vi "theta_calibration.vi"(6 "error in (no error)":errorcluster, 9 "log to file":path=path "C:/Users/tuphe10-memsbuddy/Desktop/test_VTI_theta_cal/test.txt", 11 "VISA Gaussmeter":refnum<visa-resource-name>="GPIB1::11::INSTR") -> (4 "error out":errorcluster, 5 "VISA resource name":refnum<visa-resource-name>)   [LabVIEW 2013]
uses:
  devices/gaussmeter/gaussmeter channels.ctl
panel:
  out "Channel 3":dbl format="%.2f"
  in  "channel 3":T1=enum."Z"
  out "Channel 3":cluster{dbl, dbl}[](graph)
  out "current theta (deg)":dbl format="%#_13g"
  in  "start theta (deg)":dbl format="%#_13g"
  in  "final theta (deg)":dbl=190.0 format="%#_13g"
  in  "increment (deg)":dbl=0.5 format="%#_13g"
  in  "channel 2":T1=enum."Y"
  in  "channel 1":T1
  out "Channel 2":cluster{dbl, "magnetic field (T)":dbl}[](graph)
  out "Channel 1":cluster{dbl, dbl}[](graph)
  out "Channel 2":dbl format="%.2f"
  out "Channel 1":dbl format="%.2f"
  # "This .vi sets the motor to 0deg (reference switch) & performs a user-defined turn while measuring field components with the Gaussmeter. It saves the data into a .txt file."
  # "NEVER exceed 320° !!!\nUse only positive values here!"
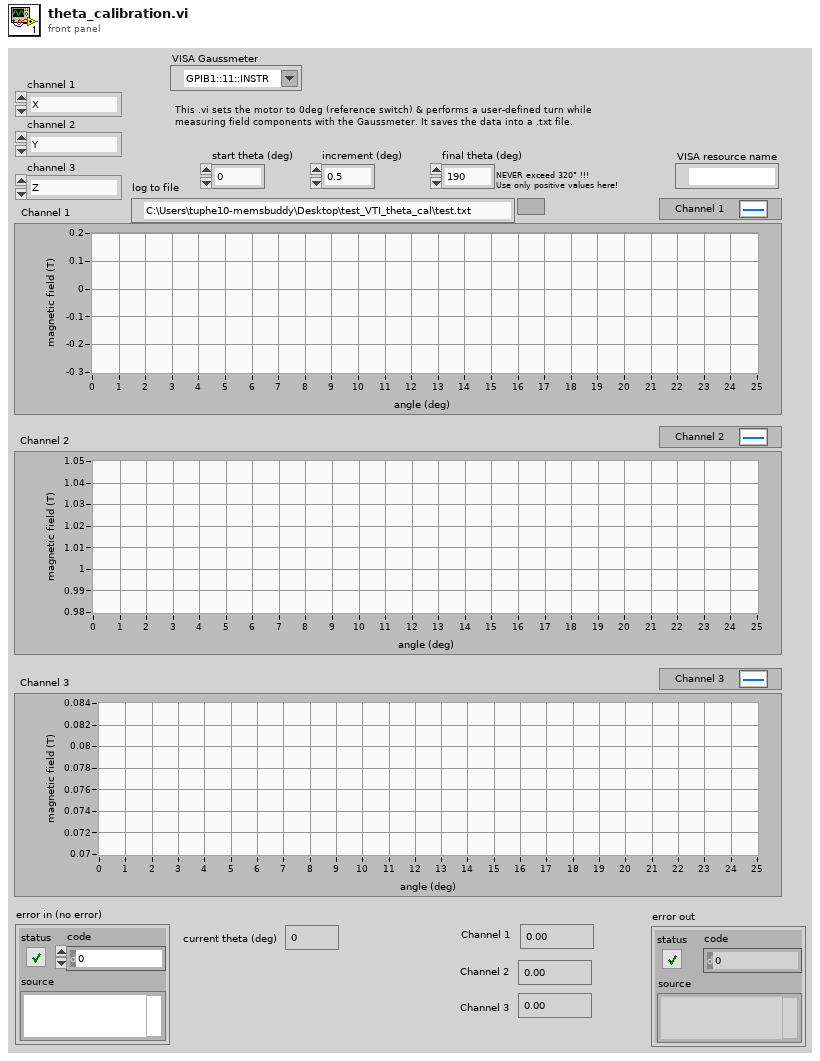
[diagram p1: front panel]
types:
  T1 = typedef "gaussmeter channels.ctl" = enum16{"X", "Y", "Z", "Vec"}
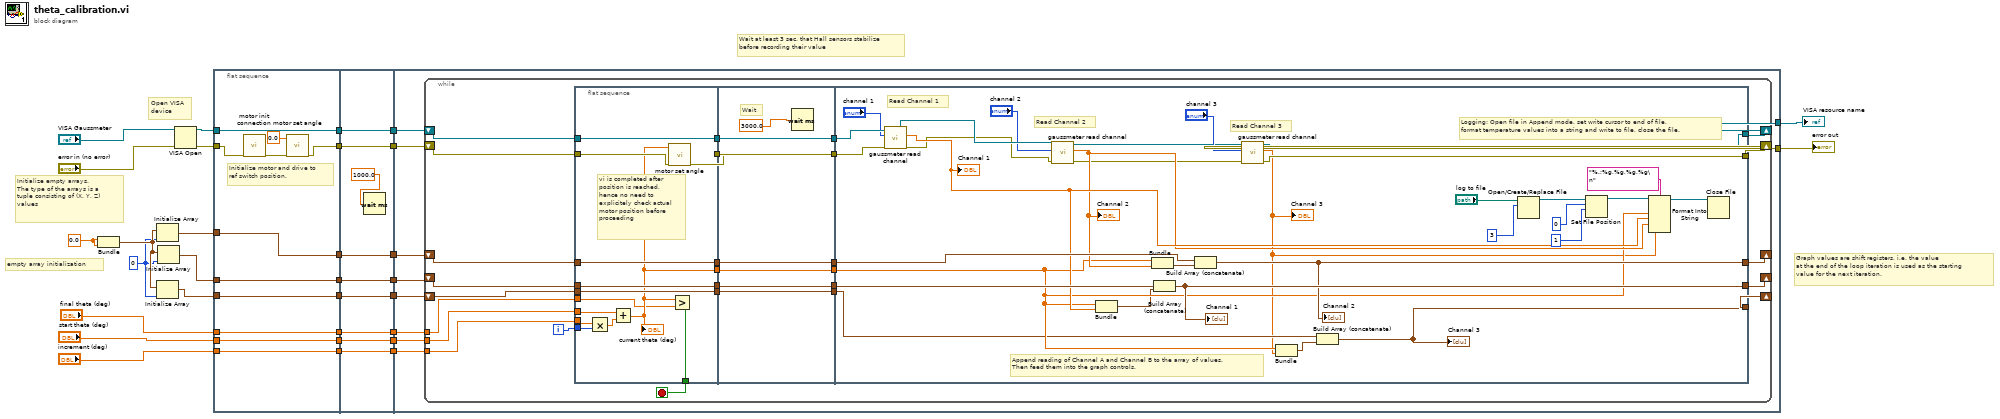
[diagram p0: block diagram]
diagram:
  w4 = 0
  w6 = 0.0
  # "Wait at least 3 sec. that Hall sensors stabilize\nbefore recording their value"
  # "empty array initialization"
  # "Graph values are shift registers, i.e. the value\nat the end of the loop iteration is used as the starting\nvalue for the next iteration."
  # "Initialize empty arrays.\nThe type of the arrays is a tuple consisting of (X, Y, Z) values"
  # "Open VISA\ndevice"
  n1 = Bundle(w6, w6) -> (w5:cluster{dbl, dbl})  [unwired: 1 in]
  n2 = Initialize Array(w5, w4) -> (w27:cluster{dbl, dbl}[])
  n3 = Initialize Array(w5, w4) -> (w2:cluster{dbl, dbl}[])
  n4 = Initialize Array(w5, w4) -> (w26:cluster{dbl, dbl}[])
  n5 = VISA Open(error in (no error)="error in (no error)", VISA resource name="VISA Gaussmeter") -> (VISA resource name=w29:refnum<visa-resource-name>, error out=w28:errorcluster)  [unwired: 3 in]
  n6 = flat-sequence {
    tunnel: "start theta (deg)" -> [w37]
    tunnel: "final theta (deg)" -> [w38]
    tunnel: "increment (deg)" -> [w39]
    tunnel: w26 -> [w40]
    tunnel: w27 -> [w41]
    tunnel: w28 -> [w34]
    tunnel: w29 -> [w42]
    tunnel: [w42] -> w20
    tunnel: [w33] -> w18
    tunnel: [w41] -> w16
    tunnel: [w40] -> w14
    tunnel: [w39] -> w12
    tunnel: [w38] -> w10
    tunnel: [w37] -> w8
    tunnel: [w32] -> w3
    tunnel: w2 -> [w32]
    tunnel: w20 -> [w51]
    tunnel: [w51] -> w19
    tunnel: w18 -> [w50]
    tunnel: [w50] -> w17
    tunnel: w16 -> [w49]
    tunnel: [w49] -> w15
    tunnel: w14 -> [w48]
    tunnel: [w48] -> w13
    tunnel: w12 -> [w47]
    tunnel: [w47] -> w11
    tunnel: w10 -> [w46]
    tunnel: [w46] -> w9
    tunnel: w8 -> [w45]
    tunnel: [w45] -> w7
    tunnel: w3 -> [w43]
    tunnel: [w43] -> w1
    tunnel: [w57] -> w25
    tunnel: [w56] -> w24
    tunnel: w19 -> [w61]
    tunnel: w17 -> [w60]
    tunnel: w15 -> [w59]
    tunnel: w13 -> [w58]
    tunnel: w11 -> [w55]
    tunnel: w9 -> [w54]
    tunnel: w7 -> [w53]
    tunnel: w1 -> [w52]
    frame #0 {
      # "Initialize motor and drive to\nref switch position."
      n7 = call "motor init connection.vi"("error in (no error)"=w34) -> ("error out"=w35:errorcluster)  [unwired: 9 in, 1 out]
      n8 = call "motor set angle.vi"("error in (no error)"=w35, "angle"=0.0) -> ("error out"=w33:errorcluster)  [unwired: 9 in]
    }
    frame #1 {
      n9 = Wait (ms)(milliseconds to wait=1000.0 ("angle")) -> ()  [unwired: 1 out]
    }
    frame #2 {
      n10 = while {
        shift-right: [w88] -> w57
        shift-left: w60 -> [w81]
        shift-right: [w87] -> w56
        shift-left: w61 -> [w82]
        shift-right: [w86] -> _
        shift-left: w58 -> [w83]
        shift-right: [w85] -> _
        shift-left: w59 -> [w84]
        tunnel: w55 -> [w78]
        tunnel: w54 -> [w76]
        tunnel: w53 -> [w77]
        shift-right: [w75] -> _
        shift-left: w52 -> [w74]
        i -> [w80]
        stop <- w79 stop-if-true
        n11 = flat-sequence {
          tunnel: w81 -> [w94]
          tunnel: w82 -> [w99]
          tunnel: w83 -> [w100]
          tunnel: w84 -> [w101]
          tunnel: [w101] -> w73
          tunnel: [w100] -> w71
          tunnel: [w99] -> w69
          tunnel: [w93] -> w67
          tunnel: [w90] -> w65
          tunnel: w80 -> [w92]
          tunnel: [w97] -> w79
          tunnel: w78 -> [w96]
          tunnel: w77 -> [w95]
          tunnel: w76 -> [w89]
          tunnel: w74 -> [w91]
          tunnel: [w91] -> w63
          tunnel: w73 -> [w108]
          tunnel: [w108] -> w72
          tunnel: w71 -> [w107]
          tunnel: [w107] -> w70
          tunnel: w69 -> [w106]
          tunnel: [w106] -> w68
          tunnel: w67 -> [w105]
          tunnel: [w105] -> w66
          tunnel: w65 -> [w104]
          tunnel: [w104] -> w64
          tunnel: w63 -> [w103]
          tunnel: [w103] -> w62
          tunnel: [w117] -> w88
          tunnel: [w116] -> w87
          tunnel: [w140] -> w86
          tunnel: [w139] -> w85
          tunnel: w72 -> [w138]
          tunnel: w70 -> [w137]
          tunnel: w68 -> [w128]
          tunnel: w66 -> [w127]
          tunnel: w64 -> [w115]
          tunnel: w62 -> [w112]
          tunnel: [w110] -> w75
          frame #0 {
            # "vi is completed after \nposition is reached, \nhence no need to \nexplicitely check actual\nmotor position before \nproceeding"
            n12 = Multiply(x=w96, y=w92) -> (x*y=w98:dbl)
            n13 = Add(x=w95, y=w98) -> (x+y=w90:dbl)
            "current theta (deg)" <- w90
            n14 = call "motor set angle.vi"("error in (no error)"=w94, "angle"=w90) -> ("error out"=w93:errorcluster)  [unwired: 9 in]
            n15 = Greater?(x=w90, y=w89) -> (0:w97:bool)
          }
          frame #1 {
            # "Wait"
            n16 = Wait (ms)(milliseconds to wait=3000.0 ("angle")) -> ()  [unwired: 1 out]
          }
          frame #2 {
            # "Read Channel 3"
            # "Logging: Open file in Append mode, set write cursor to end of file,\nformat temperature values into a string and write to file, close the file."
            # "Append reading of Channel A and Channel B to the array of values.\nThen feed them into the graph controls."
            # "Read Channel 2"
            # "Read Channel 1"
            n17 = call "gaussmeter read channel.vi"("error in (no error)"=w127, "channel"="channel 1", "VISA resource name"=w128) -> ("error out"=w123:errorcluster, "magnetic field (T)"=w125:dbl, "VISA resource name 2"=w124:refnum<visa-resource-name>)  [unwired: 6 in]
            "Channel 1" <- w125
            n18 = call "gaussmeter read channel.vi"("error in (no error)"=w123, "channel"="channel 2", "VISA resource name"=w124) -> ("error out"=w118:errorcluster, "magnetic field (T)"=w121:dbl, "VISA resource name 2"=w119:refnum<visa-resource-name>)  [unwired: 6 in]
            "Channel 2" <- w121
            n19 = Bundle(w115, "magnetic field (T)"=w125) -> (w113:cluster{dbl, "magnetic field (T)":dbl})  [unwired: 1 in]
            n20 = Bundle(w115, "magnetic field (T)"=w121) -> (w114:cluster{dbl, "magnetic field (T)":dbl})  [unwired: 1 in]
            n21 = Build Array (concatenate)(w137, w113) -> (w140:cluster{dbl, "magnetic field (T)":dbl}[])
            "Channel 1" <- w140
            n22 = Build Array (concatenate)(w138, w114) -> (w139:cluster{dbl, "magnetic field (T)":dbl}[])
            "Channel 2" <- w139
            n23 = call "gaussmeter read channel.vi"("error in (no error)"=w118, "channel"="channel 3", "VISA resource name"=w119) -> ("error out"=w117:errorcluster, "magnetic field (T)"=w109:dbl, "VISA resource name 2"=w116:refnum<visa-resource-name>)  [unwired: 6 in]
            "Channel 3" <- w109
            n24 = Bundle(w115, "magnetic field (T)"=w109) -> (w111:cluster{dbl, "magnetic field (T)":dbl})  [unwired: 1 in]
            n25 = Build Array (concatenate)(w112, w111) -> (w110:cluster{dbl, "magnetic field (T)":dbl}[])
            "Channel 3" <- w110
            n26 = Open/Create/Replace File(file path (use dialog)="log to file", operation (0:open)=3) -> (refnum out=w134:refnum<file>)  [unwired: 4 in, 2 out]
            n27 = Set File Position(offset (in bytes) (0)=0, refnum=w134, from (0:start)=1) -> (refnum out=w133:refnum<file>)  [unwired: 1 in, 1 out]
            n28 = Format Into String(format string="%.;%g,%g,%g,%g\n", initial string=w133, w115, w125, w121, w109) -> (resulting string=w132:refnum<file>)  [unwired: 1 in, 1 out]
            n29 = Close File(refnum=w132) -> ()  [unwired: 1 in, 2 out]
          }
        }
      }
    }
  }
  "error out" <- w25
  "VISA resource name" <- w24
